vi "SectorEdgeTestCompile.vi"   [LabVIEW 2013]
uses:
  <vilib>/rvi/DataTransferAndStorage/Container/XNode/niFpgaContainer.xnode
  <vilib>/rvi/FIFO/Fifo_Resource/nirvififoEmulationWrite.vi
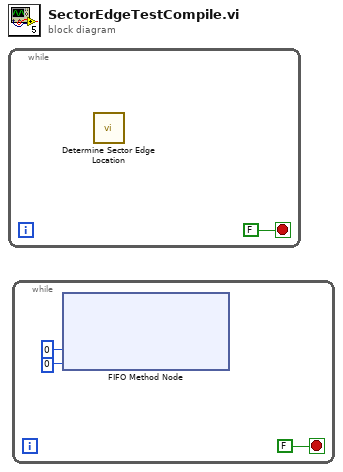
[diagram p0: block diagram]
diagram:
  n1 = while {
    stop <- FALSE stop-if-true
    n2 = call "Determine Sector Edge Location.vi"() -> ()  [unwired: 10 in, 2 out]
  }
  n3 = while {
    stop <- FALSE stop-if-true
    n4 = xnode ("FIFO Method Node")("Element"=u8 0, "Timeout"=0) -> ()  [unwired: 1 in, 2 out]
  }
